vi "PEAK_Can_Read.vi"(8 "errin":errorcluster, 11 "Channel out":T2) -> (0 "errout":errorcluster, 2 "TimestampBuffer out 2":T1, 3 "MessageBuffer out":T3)   [LabVIEW 2020, in "PEAK_lib_ALEX.lvlib"]
uses:
  <userlib>/Alex_Peak_lib/PEAK_lib_ALEX.lvlib
  <vilib>/Sylvain.lib/user.lib/PCAN Basic/Controls/Channel.ctl
  PCANBasic.dll
  <userlib>/PCAN Basic/PCANBasic.lvlib
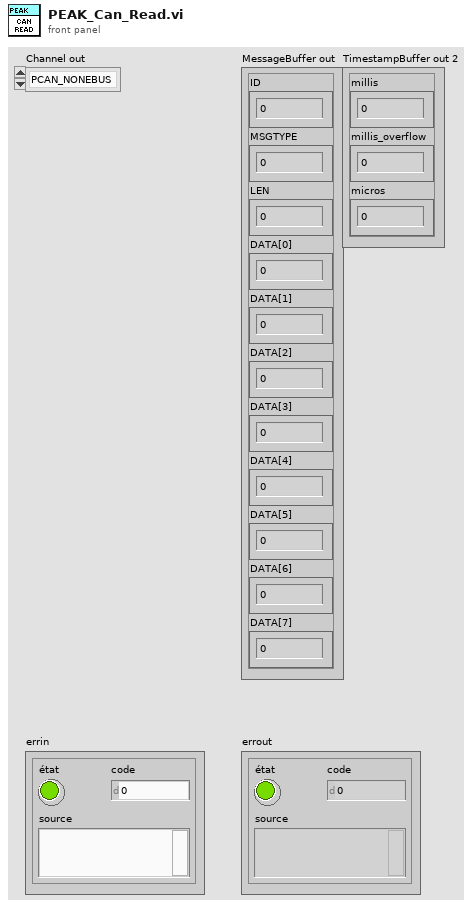
[diagram p1: front panel]
types:
  T1 = cluster{"millis":u32, "millis_overflow":u16, "micros":u16}
  T2 = typedef "PCANBasic.lvlib/Channel.ctl" = enum16{"PCAN_NONEBUS", "not used1", "not used2", "not used3", "not used4", "not used5", "not used6", "not used7", "not used8", "not used9", "not used10", "not used11", "not used12", "not used13", "not used14", "not used15", "not used16", "not used17", "not used18", "not used19", "not used20", "not used21", "not used22", "not used23", "not used24", "not used25", "not used26", "not used27", "not used28", "not used29", "not used30", "not used31", "not used32", "PCAN_ISABUS1", "PCAN_ISABUS2", "PCAN_ISABUS3", "PCAN_ISABUS4", "PCAN_ISABUS5", "PCAN_ISABUS6", "PCAN_ISABUS7", "PCAN_ISABUS8", "not used41", "not used42", "not used43", "not used44", "not used45", "not used46", "not used47", "not used48", "PCAN_DNGBUS1", "not used50", "not used51", "not used52", "not used53", "not used54", "not used55", "not used56", "not used57", "not used58", "not used59", "not used60", "not used61", "not used62", "not used63", "not used64", "PCAN_PCIBUS1", "PCAN_PCIBUS2", "PCAN_PCIBUS3", "PCAN_PCIBUS4", "PCAN_PCIBUS5", "PCAN_PCIBUS6", "PCAN_PCIBUS7", "PCAN_PCIBUS8", "not used73", "not used74", "not used75", "not used76", "not used77", "not used78", "not used79", "not used80", "PCAN_USBBUS1", "PCAN_USBBUS2", "PCAN_USBBUS3", "PCAN_USBBUS4", "PCAN_USBBUS5", "PCAN_USBBUS6", "PCAN_USBBUS7", "PCAN_USBBUS8", "Not used89", "Not used90", "Not used91", "Not used92", "Not used93", "Not used94", "Not used95", "Not used96", "PCAN_PCCBUS1", "PCAN_PCCBUS2"}
  T3 = cluster{"ID":u32, "MSGTYPE":u8, "LEN":u8, "DATA[0]":u8, "DATA[1]":u8, "DATA[2]":u8, "DATA[3]":u8, "DATA[4]":u8, "DATA[5]":u8, "DATA[6]":u8, "DATA[7]":u8}
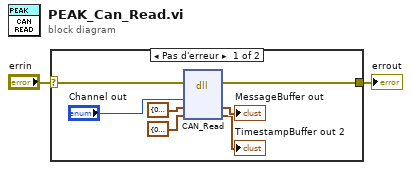
[diagram p0: block diagram]
diagram:
  n1 = case shown="Pas d'erreur" "errin" {
    selector: "errin" -> [w4 w10]
    tunnel: [w9 w10] -> w2
    frame No Error {
      n2 = dll-call lib="PCANBasic.dll" fn="CAN_Read"(error in=w4, "Channel"="Channel out", "MessageBuffer"=T3 {"ID"=0, "MSGTYPE"=0, "LEN"=0, "DATA[0]"=0, "DATA[1]"=0, "DATA[2]"=0, "DATA[3]"=0, "DATA[4]"=0, "DATA[5]"=0, "DATA[6]"=0, "DATA[7]"=0} ("MessageBuffer out"), "TimestampBuffer"=T1 {"millis"=0, "millis_overflow"=0, "micros"=0} ("TimestampBuffer out 2")) -> (error out=w9:errorcluster, "MessageBuffer"=→"MessageBuffer out":T3, "TimestampBuffer"=→"TimestampBuffer out 2":T1)  [unwired: 4 in, 1 out]
    }
    frame Error {
    }
  }
  "errout" <- w2
